vi "04-MatchNumber.vi"() -> ()   [LabVIEW 2014]
panel:
  out "# interactions":dbl
  out "Current number":dbl
  in  "Number to match":dbl
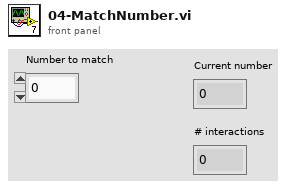
[diagram p1: front panel]
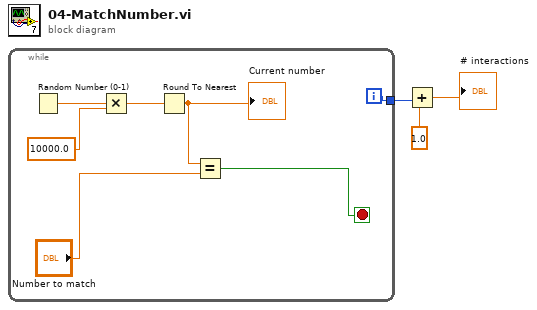
[diagram p0: block diagram]
diagram:
  n1 = while {
    tunnel: [w7] -> w2
    i -> [w7]
    stop <- w4 stop-if-true
    n2 = Random Number (0-1)() -> (number: 0 to 1=w10:dbl)
    n3 = Multiply(x=w10, y=10000.0 ("x*y")) -> (x*y=w8:dbl)
    n4 = Round To Nearest(number=w8) -> (nearest integer value=w6:dbl)
    "Current number" <- w6
    n5 = Equal?(x=w6, y="Number to match") -> (x = y?=w4:bool)
  }
  n6 = Add(x=1.0, y=w2) -> (x+y=→"# interactions":dbl)
